vi "TearDown.vi"(8 "error in (no error)":errorcluster, 11 "BuildManager in":refnum<class "BuildManager.lvclass">) -> (0 "error out":errorcluster, 3 "BuildManager out":refnum<class "BuildManager.lvclass">)   [LabVIEW 2019, in "SolutionBuilder.lvlib" / "BuildManager.lvclass"]
uses:
  BuildManager.lvclass
  GeneratedFile.ctl
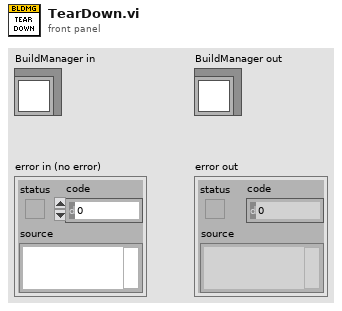
[diagram p1: front panel]
types:
  T1 = typedef "SolutionBuilder.lvlib/BuildManager.lvclass/GeneratedFile.ctl" = map{cluster{"Project path":path, "Build spec name":string}, set{path}}
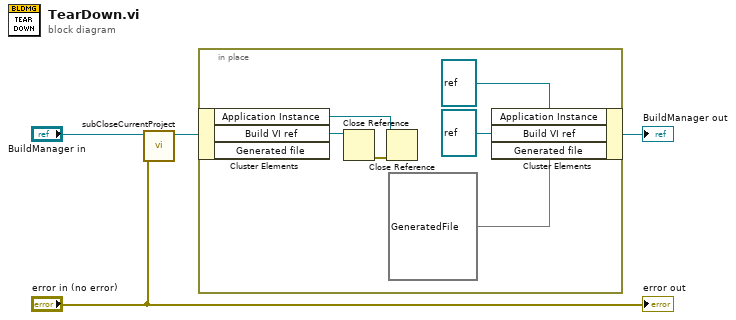
[diagram p0: block diagram]
diagram:
  n1 = call "subCloseCurrentProject.vi"("error in (no error)"="error in (no error)", "BuildManager in"="BuildManager in") -> ("BuildManager out"=w3:refnum<class "BuildManager.lvclass">)  [unwired: 8 in, 1 out]
  n2 = in-place {
    n3 = in-place-cluster #1(w3) -> ("Application Instance"=w7:refnum<vi>, "Build VI ref"=w10:refnum<vi>)  [unwired: 1 out]
    n4 = Close Reference(reference=w10) -> (error out=w8:errorcluster)  [unwired: 1 in]
    n5 = Close Reference(reference=w7, error in (no error)=w8) -> ()  [unwired: 1 out]
    n6 = in-place-cluster #1("Application Instance"=refnum<vi> refnum, "Build VI ref"=refnum<vi> refnum, "Generated file"=T1 {}) -> (→"BuildManager out":refnum<class "BuildManager.lvclass">)
  }
  "error out" <- "error in (no error)"
